vi "Complete Call.vi"(0 "gRPCid":T1, 3 "error in":errorcluster) -> (10 "error out":errorcluster)   [LabVIEW 2019, in "grpc-lvsupport.lvlib"]
uses:
  grpc-lvsupport.lvlib
  Shared/grpcId.ctl
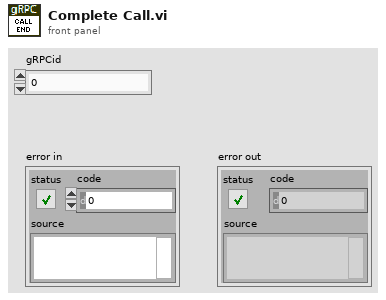
[diagram p1: front panel]
types:
  T1 = typedef "grpc-lvsupport.lvlib/grpcId.ctl" = u64
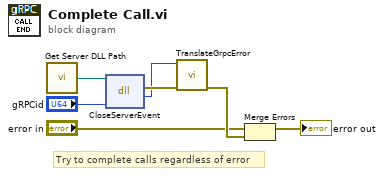
[diagram p0: block diagram]
diagram:
  # "Try to complete calls regardless of error"
  n1 = call "Get Server DLL Path.vi"() -> ("Server dll path"=w5:path)
  n2 = dll-call lib="C:/Users/XEnderMD/Desktop/LV gRPC/labview source/gRPC interface/dlls/labview_grpc_server.dll" fn="CloseServerEvent"(path in=w5, "id"="gRPCid") -> (error out=w7:errorcluster, "return type"=w3:i32)  [unwired: 3 in, 1 out]
  n3 = call "TranslateGrpcError.vi"("error in"=w7, "Error Code"=w3) -> ("error out"=w4:errorcluster)  [unwired: 9 in]
  n4 = Merge Errors("error in", w4) -> (→"error out":errorcluster)
